vi "StackingClassifier.vi"(8 "error in":errorcluster) -> (0 "error out":errorcluster, 3 "out":refnum<class "StackingClassifier.lvclass">)   [LabVIEW 2020]
doc: "Stack of estimators with a final classifier.\n\n Stacked generalization consists in stacking the output of individual\n estimator and use a classifier to compute the final prediction. Stacking\n allows to use the strength of each individual estimator by using their\n output as input of a final estimator.\n\n Note that `estimators_` are fitted on the full `X` while `final_estimator_`\n is trained using cross-validated predictions of the base estimators using\n `cross_val_predict`.\n\n Read more in the :ref:`User Guide <stacking>`.\n\n .. versionadded:: 0.22\n\n Parameters\n ----------\n estimators : list of (str, estimator)\n Base estimators which will be stacked together. Each element of the\n list is defined as a tuple of string (i.e. name) and an estimator\n instance. An estimator can be set to 'drop' using `set_params`.\n\n final_estimator : estimator, default=None\n A classifier which will be used to combine the base estimators.\n The default classifier is a\n :class:`~sklearn.linear_model.LogisticRegression`.\n\n cv : int, cross-validation generator or an iterable, default=None\n Determines the cross-validation splitting strategy used in\n `cross_val_predict` to train `final_estimator`. Possible inputs for\n cv are:\n\n * None, to use the default 5-fold cross validation,\n * integer, to specify the number of folds in a (Stratified) KFold,\n * An object to be used as a cross-validation generator,\n * An iterable yielding train, test splits.\n\n For integer/None inputs, if the estimator is a classifier and y is\n either binary or multiclass,\n :class:`~sklearn.model_selection.StratifiedKFold` is used.\n In all other cases, :class:`~sklearn.model_selection.KFold` is used.\n These splitters are instantiated with `shuffle=False` so the splits\n will be the same across calls.\n\n Refer :ref:`User Guide <cross_validation>` for the various\n cross-validation strategies that can be used here.\n\n .. note::\n A larger number of split will provide no benefits if the number\n of training samples is large enough. Indeed, the training time\n will increase. ``cv`` is not used for model evaluation but for\n prediction.\n\n stack_method : {'auto', 'predict_proba', 'decision_function', 'predict'}, default='auto'\n Methods called for each base estimator. It can be:\n\n * if 'auto', it will try to invoke, for each estimator,\n `'predict_proba'`, `'decision_function'` or `'predict'` in that\n order.\n * otherwise, one of `'predict_proba'`, `'decision_function'` or\n `'predict'`. If the method is not implemented by the estimator, it\n will raise an error.\n\n n_jobs : int, default=None\n The number of jobs to run in parallel all `estimators` `fit`.\n `None` means 1 unless in a `joblib.parallel_backend` context. -1 means\n using all processors. See Glossary for more details.\n\n passthrough : bool, default=False\n When False, only the predictions of estimators will be used as\n training data for `final_estimator`. When True, the\n `final_estimator` is trained on the predictions as well as the\n original training data.\n\n verbose : int, default=0\n Verbosity level.\n\n Attributes\n ----------\n classes_ : ndarray of shape (n_classes,)\n Class labels.\n\n estimators_ : list of estimators\n The elements of the estimators parameter, having been fitted on the\n training data. If an estimator has been set to `'drop'`, it\n will not appear in `estimators_`.\n\n named_estimators_ : :class:`~sklearn.utils.Bunch`\n Attribute to access any fitted sub-estimators by name.\n\n final_estimator_ : estimator\n The classifier which predicts given the output of `estimators_`.\n\n stack_method_ : list of str\n The method used by each base estimator.\n\n Notes\n -----\n When `predict_proba` is used by each estimator (i.e. most of the time for\n `stack_method='auto'` or specifically for `stack_method='predict_proba'`),\n The first column predicted by each estimator will be dropped in the case\n of a binary classification problem. Indeed, both feature will be perfectly\n collinear.\n\n References\n ----------\n .. [1] Wolpert, David H. \"Stacked generalization.\" Neural networks 5.2\n (1992): 241-259.\n\n \nAvailable methods:\nFit Transform\nTransform\nFit\nPredict\nScore\nGet Attributes\nGet Params\nSet Params"
uses:
  StackingClassifier.lvclass
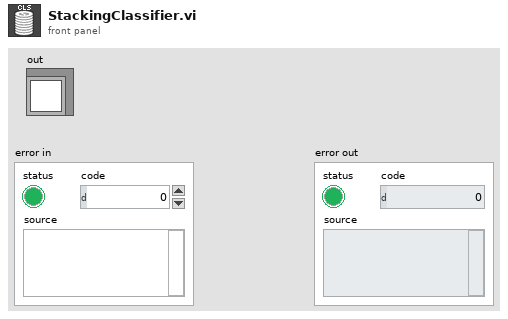
[diagram p1: front panel]
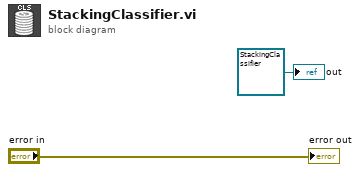
[diagram p0: block diagram]
diagram:
  "out" <- refnum<class "StackingClassifier.lvclass"> refnum ("model")
  "error out" <- "error in"
